vi "fileInput.vi"(5 "basePath in":string, 6 "pathList in":string[](array[string]), 7 "Type and Defaults in":variant, 8 "error in (no error)":errorcluster, 9 "String in":string, 10 "json file?":bool, 11 "file (use dialog)":path) -> (0 "error out":errorcluster, 1 "basePath out":string, 2 "String out":string, 3 "Type and Defaults out":variant, 4 "pathList out":string[](array[string]))   [LabVIEW 2015]
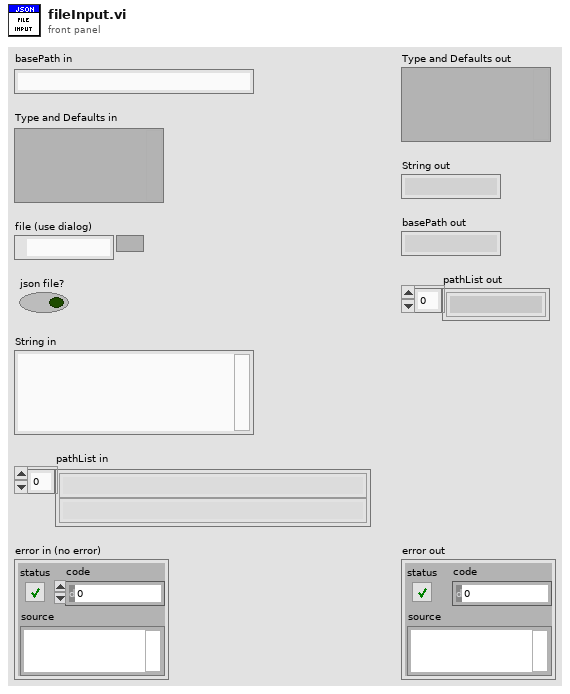
[diagram p1: front panel]
types:
  T1 = enum16{"open", "replace", "create", "open or create", "replace or create", "replace or create with confirmation"}
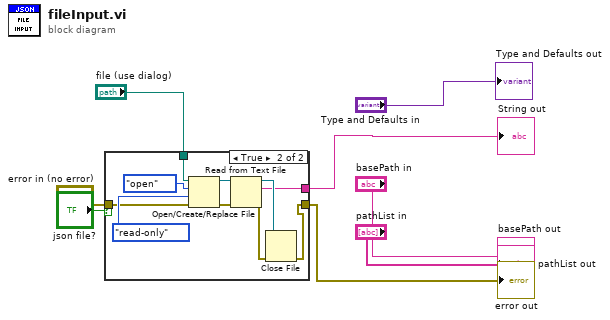
[diagram p0: block diagram]
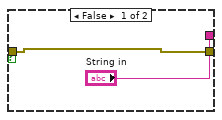
[diagram p2: hidden frame]
diagram:
  n1 = case shown="True" "json file?" {
    tunnel: ["String in" w11] -> w4
    tunnel: "file (use dialog)" -> [_ w18]
    tunnel: [w9 w12] -> w5
    tunnel: "error in (no error)" -> [w9 w15]
    frame False {
    }
    frame True {
      n2 = Open/Create/Replace File(file path (use dialog)=w18, error in=w15, operation (0:open)=T1."open", access (0:read/write)=enum16{"read/write", "read-only", "write-only"}."read-only") -> (refnum out=w17:refnum<file>, error out=w16:errorcluster)  [unwired: 2 in, 1 out]
      n3 = Read from Text File(file (use dialog)=w17, error in=w16) -> (refnum out=w14:refnum<file>, text=w11:string, error out=w13:errorcluster)  [unwired: 2 in, 1 out]
      n4 = Close File(refnum=w14, error in=w13) -> (error out=w12:errorcluster)  [unwired: 1 out]
    }
  }
  "error out" <- w5
  "String out" <- w4
  "pathList out" <- "pathList in"
  "basePath out" <- "basePath in"
  "Type and Defaults out" <- "Type and Defaults in"
